vi "sensor.vi"(3 "Sensor":string) -> (0 "2":bool, 1 "1":bool)   [LabVIEW 2023]
uses:
  <vilib>/DAQmx/read.llb/DAQmx Read (Digital Bool 1Line 1Point).vi
  <vilib>/DAQmx/create/channels.llb/DAQmx Create Channel (DI-Digital Input).vi
  <vilib>/DAQmx/miscellaneous.llb/DAQmx Fill In Error Info.vi
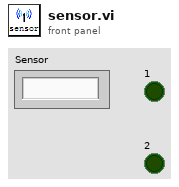
[diagram p1: front panel]
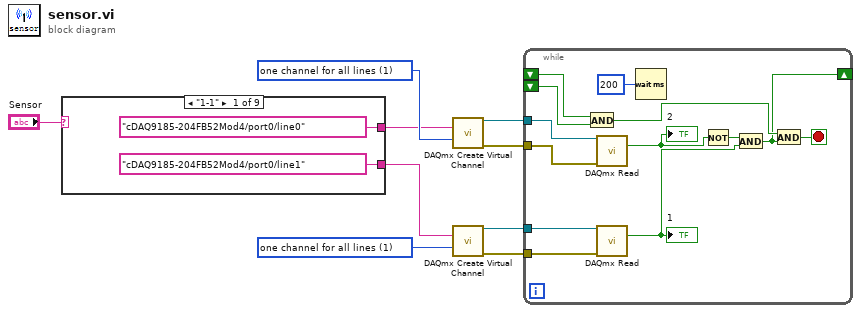
[diagram p0: block diagram]
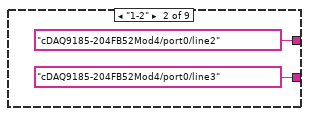
[diagram p2: hidden frame]
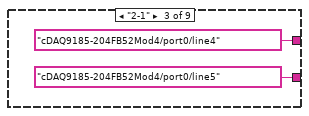
[diagram p3: hidden frame]
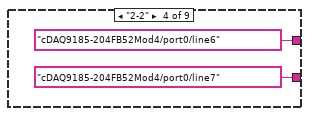
[diagram p4: hidden frame]
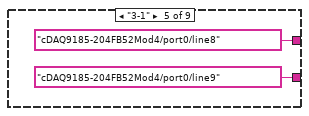
[diagram p5: hidden frame]
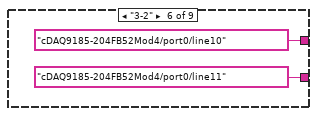
[diagram p6: hidden frame]
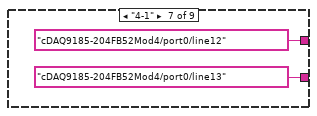
[diagram p7: hidden frame]
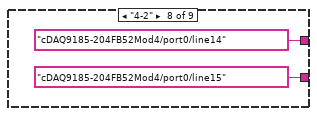
[diagram p8: hidden frame]
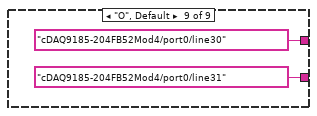
[diagram p9: hidden frame]
diagram:
  w4 = 1 items=["one channel for each line", "one channel for all lines"] ("line grouping")
  w5 = 1 items=["one channel for each line", "one channel for all lines"] ("line grouping")
  n1 = case shown="\"1-1\"" "Sensor" {
    tunnel: [tag "cDAQ9185-204FB52Mod4/port0/line0" ("lines") tag "cDAQ9185-204FB52Mod4/port0/line2" ("lines") tag "cDAQ9185-204FB52Mod4/port0/line4" ("lines") tag "cDAQ9185-204FB52Mod4/port0/line6" ("lines") tag "cDAQ9185-204FB52Mod4/port0/line8" ("lines") tag "cDAQ9185-204FB52Mod4/port0/line10" ("lines") tag "cDAQ9185-204FB52Mod4/port0/line12" ("lines") tag "cDAQ9185-204FB52Mod4/port0/line14" ("lines") tag "cDAQ9185-204FB52Mod4/port0/line30" ("lines")] -> w3
    tunnel: [tag "cDAQ9185-204FB52Mod4/port0/line1" ("lines") tag "cDAQ9185-204FB52Mod4/port0/line3" ("lines") tag "cDAQ9185-204FB52Mod4/port0/line5" ("lines") tag "cDAQ9185-204FB52Mod4/port0/line7" ("lines") tag "cDAQ9185-204FB52Mod4/port0/line9" ("lines") tag "cDAQ9185-204FB52Mod4/port0/line11" ("lines") tag "cDAQ9185-204FB52Mod4/port0/line13" ("lines") tag "cDAQ9185-204FB52Mod4/port0/line15" ("lines") tag "cDAQ9185-204FB52Mod4/port0/line31" ("lines")] -> w2
    frame "1-1" {
    }
    frame "1-2" {
    }
    frame "2-1" {
    }
    frame "2-2" {
    }
    frame "3-1" {
    }
    frame "3-2" {
    }
    frame "4-1" {
    }
    frame "4-2" {
    }
    frame "O", Default {
    }
  }
  n2 = call-poly <vilib>:"DAQmx Create Virtual Channel.vi"("lines"=w3, "line grouping"=w4) -> ("task out"=w8:refnum<k21>, "error out"=w9:errorcluster)  [unwired: 12 in]
  n3 = call-poly <vilib>:"DAQmx Create Virtual Channel.vi"("lines"=w2, "line grouping"=w5) -> ("task out"=w6:refnum<k21>, "error out"=w7:errorcluster)  [unwired: 12 in]
  n4 = while {
    tunnel: w6 -> [w40]
    tunnel: w7 -> [w39]
    tunnel: w8 -> [w38]
    tunnel: w9 -> [w37]
    shift-right: [w30] -> _
    shift-left: _ -> [w33]
    shift-left: _ -> [w32]
    stop <- w29 stop-if-true
    n5 = And(x=w33, y=w32) -> (x .and. y?=w31:bool)
    n6 = call-poly <vilib>:"DAQmx Read.vi"("task/channels in"=w38, "error in"=w37) -> ("data"=w36:bool)  [unwired: 11 in, 2 out]
    "2" <- w36
    n7 = call-poly <vilib>:"DAQmx Read.vi"("task/channels in"=w40, "error in"=w39) -> ("data"=w34:bool)  [unwired: 11 in, 2 out]
    "1" <- w34
    n8 = Wait (ms)(milliseconds to wait=u32 200) -> ()  [unwired: 1 out]
    n9 = Not(x=w36) -> (.not. x?=w35:bool)
    n10 = And(x=w35, y=w34) -> (x .and. y?=w30:bool)
    n11 = And(x=w31, y=w30) -> (x .and. y?=w29:bool)
  }
